vi "Test Does not Append nn color.vi"(11 "Test Case In":refnum<class "Added Section Finder Test.lvclass">) -> (0 "error out":errorcluster, 3 "Test Case Out":refnum<class "Added Section Finder Test.lvclass">)   [LabVIEW 2020, in "Added Section Finder Test.lvclass"]
uses:
  Added Section Finder Test.lvclass
  usr/local/natinst/LabVIEW-2026-64/vi.lib/Astemes/LUnit/Test Case.lvclass
  <vilib>/Astemes/LUnit/Test Case.lvclass/Test Case.ctl
  06a737ec-4e69-4fba-9170-4fe28b1e630c.vi
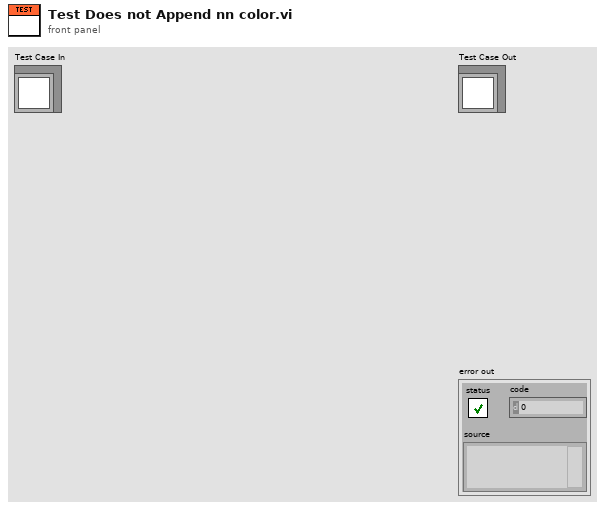
[diagram p1: front panel]
types:
  T1 = cluster{"Selection Start":u32, "Selection End":u32}[]
  T2 = cluster{"Selection Start":u32, "Selection End":u32}
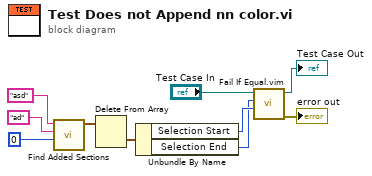
[diagram p0: block diagram]
diagram:
  n1 = call "Find Added Sections.vi"("Offset"=u32 0 ("Index"), "Reference"="ad", "Target"="asd") -> ("Sections in Target"=w7:T1)  [unwired: 8 in]
  n2 = Delete From Array(array=w7) -> (deleted portion=w6:T2)  [unwired: 2 in, 1 out]
  n3 = Unbundle By Name(w6) -> ("Selection Start"=w3:u32, "Selection End"=w2:u32)
  n4 = call "Fail If Equal.vim"("Actual"=w3, "Unexpected"=w2, "LUnit Test Case In"="Test Case In") -> ("error out"=→"error out":errorcluster, "LUnit Test Case Out"=→"Test Case Out":refnum<class "Added Section Finder Test.lvclass">)  [unwired: 7 in]
